vi "Apply Precision to loaded file.vi"(8 "CMD Step":dbl format="%#_13g", 9 "Stats In":string[][](array[string]), 11 "Data In":string[][](array[string])) -> (1 "Stats Out":string[][](array[string]), 3 "Data Out":string[][](array[string]))   [LabVIEW 2019]
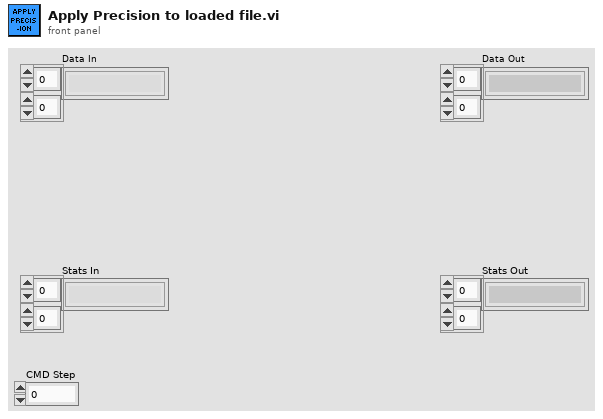
[diagram p1: front panel]
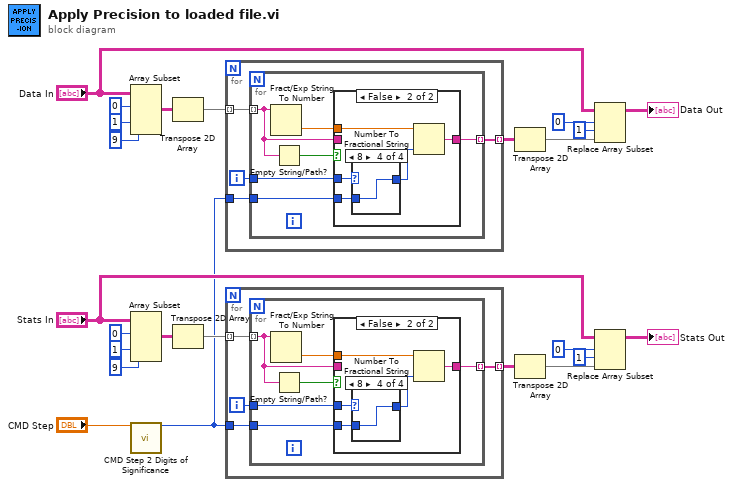
[diagram p0: block diagram]
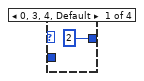
[diagram p3: hidden frame]
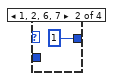
[diagram p4: hidden frame]
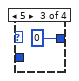
[diagram p5: hidden frame]
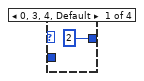
[diagram p7: hidden frame]
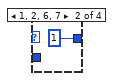
[diagram p8: hidden frame]
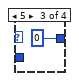
[diagram p9: hidden frame]
diagram:
  n1 = Array Subset(array="Data In", index (row)=0 ("index"), index (col)=1 ("index"), length (col)=9 ("length")) -> (w10:string[][])  [unwired: 1 in]
  n2 = Array Subset(array="Stats In", index (row)=0 ("index"), index (col)=1 ("index"), length (col)=9 ("length")) -> (w20:string[][])  [unwired: 1 in]
  n3 = call "CMD Step 2 Digits of Significance.vi"("CMD Step"="CMD Step") -> ("Digits of Significance"=w1:i32)  [unwired: 14 in]
  n4 = Transpose 2D Array(2D array=w10) -> (transposed array=w3:string[][])
  n5 = Transpose 2D Array(2D array=w20) -> (transposed array=w14:string[][])
  n6 = for {
    tunnel: [w28] -> w2 mode=indexing
    tunnel: w3 -> [w27] mode=indexing
    tunnel: w1 -> [w25]
    i -> [w26]
    n7 = for {
      tunnel: [w34] -> w28 mode=indexing
      tunnel: w27 -> [w31] mode=indexing
      tunnel: w26 -> [w30]
      tunnel: w25 -> [w29]
      n8 = Fract/Exp String To Number(string=w31) -> (number=w33:dbl)  [unwired: 3 in, 1 out]
      n9 = Empty String/Path?(string/path=w31) -> (empty?=w32:bool)
      n10 = case shown="False" w32 {
        tunnel: [w35 w40] -> w34
        tunnel: w30 -> [_ w38]
        tunnel: w33 -> [_ w37]
        tunnel: w31 -> [w35 _]
        tunnel: w29 -> [_ w36]
        frame True {
        }
        frame False {
          n11 = case shown="8" w38 {
            tunnel: [2 1 0 w44] -> w39
            tunnel: w36 -> [_ _ _ w44]
            frame 0, 3, 4, Default {
            }
            frame 1, 2, 6, 7 {
            }
            frame 5 {
            }
            frame 8 {
            }
          }
          n12 = Number To Fractional String(number=w37, precision (6)=w39) -> (F-format string=w40:string)  [unwired: 2 in]
        }
      }
    }
  }
  n13 = for {
    tunnel: [w48] -> w21 mode=indexing
    tunnel: w14 -> [w47] mode=indexing
    tunnel: w1 -> [w45]
    i -> [w46]
    n14 = for {
      tunnel: [w54] -> w48 mode=indexing
      tunnel: w47 -> [w51] mode=indexing
      tunnel: w46 -> [w50]
      tunnel: w45 -> [w49]
      n15 = Fract/Exp String To Number(string=w51) -> (number=w53:dbl)  [unwired: 3 in, 1 out]
      n16 = Empty String/Path?(string/path=w51) -> (empty?=w52:bool)
      n17 = case shown="False" w52 {
        tunnel: [w55 w60] -> w54
        tunnel: w50 -> [_ w58]
        tunnel: w53 -> [_ w57]
        tunnel: w51 -> [w55 _]
        tunnel: w49 -> [_ w56]
        frame True {
        }
        frame False {
          n18 = case shown="8" w58 {
            tunnel: [2 1 0 w64] -> w59
            tunnel: w56 -> [_ _ _ w64]
            frame 0, 3, 4, Default {
            }
            frame 1, 2, 6, 7 {
            }
            frame 5 {
            }
            frame 8 {
            }
          }
          n19 = Number To Fractional String(number=w57, precision (6)=w59) -> (F-format string=w60:string)  [unwired: 2 in]
        }
      }
    }
  }
  n20 = Transpose 2D Array(2D array=w2) -> (transposed array=w9:string[][])
  n21 = Transpose 2D Array(2D array=w21) -> (transposed array=w22:string[][])
  n22 = Replace Array Subset(array="Data In", new element=w9, index (row)=0 ("disabled index (row)"), index (col)=1 ("disabled index (col)")) -> (→"Data Out":string[][])
  n23 = Replace Array Subset(array="Stats In", new element=w22, index (row)=0 ("disabled index (row)"), index (col)=1 ("disabled index (col)")) -> (→"Stats Out":string[][])
